vi "Set Frame to send.vi"(8 "error in (no error)":errorcluster caption="entrée d'erreur (pas d'erreur)", 10 "Frame to send":string, 11 "Parsing Data (Default) en entrée":refnum<class "Parsing Frame (Default).lvclass">) -> (0 "error out":errorcluster caption="sortie d'erreur", 3 "Parsing Data (Default) en sortie":refnum<class "Parsing Frame (Default).lvclass">)   [LabVIEW 2020, in "Library Instrument & Equipement.lvlib" / "Library UART.lvlib" / "Parsing Frame (Default).lvclass"]
uses:
  Parsing Frame (Default).lvclass
  Parsing Frame (Default).lvclass/Parsing Frame (Default).ctl
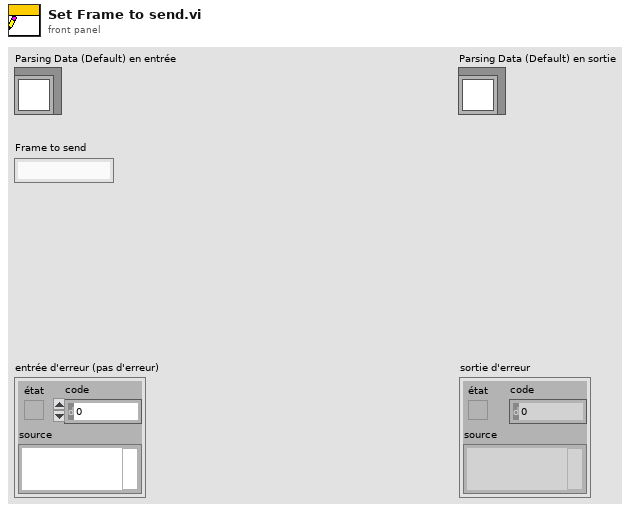
[diagram p1: front panel]
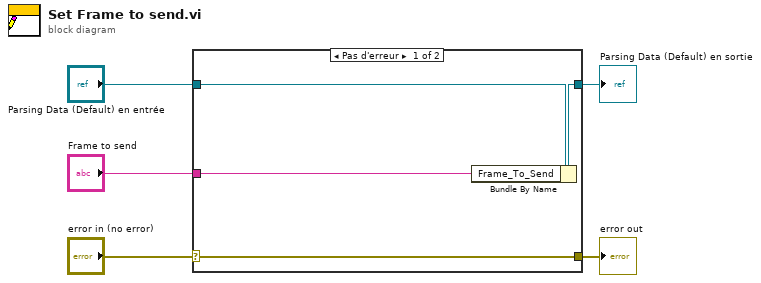
[diagram p0: block diagram]
diagram:
  n1 = case shown="Pas d'erreur" "error in (no error)" {
    selector: "error in (no error)" -> [w9 w10]
    tunnel: [w9 w10] -> w4
    tunnel: [w7 w11] -> w2
    tunnel: "Parsing Data (Default) en entrée" -> [w8 w11]
    tunnel: "Frame to send" -> [w6 _]
    frame No Error {
      n2 = Bundle By Name(cluster=w8, "Frame_To_Send"=w6) -> (w7:refnum<class "Parsing Frame (Default).lvclass">)
    }
    frame Error {
    }
  }
  "error out" <- w4
  "Parsing Data (Default) en sortie" <- w2
